vi "Compare.vi"() -> ()   [LabVIEW 2014]
doc: "Use this template to build a VI to use as a subVI."
uses:
  <vilib>/vision/NI_Vision_Development_Module.lvlib
panel:
  out "SrcA":T1(plugin-control)
  out "Dst":T1(plugin-control)
  # ":: MVi Framework V1.0 ::\nAuthor:Gaoke Yang\nEmail: gaoke.yang@yahoo.com\nWeb: www.mvicontrol.com\nCopyright (C) 2015, MVI Technologies All Rights Reserved"
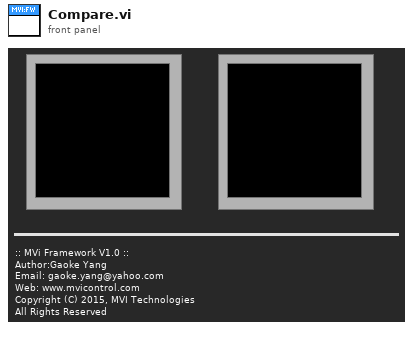
[diagram p1: front panel]
types:
  T1 = typedef "IMAQ Image.ctl" = refnum<image>
  T2 = typedef "Image Type" = u32
  T3 = enum32{"Average", "Min", "Max", "Clear  if < ", "Clear  if < or =", "Clear  if =", "Clear  if > or =", "Clear  if >"}
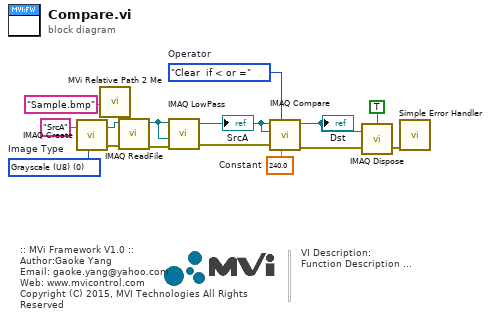
[diagram p0: block diagram]
diagram:
  w1 = T2 0 items=["Grayscale (U8)", "Grayscale (I16)", "Grayscale (SGL)", "Complex (CSG)", "RGB (U32)", "HSL (U32)", "RGB (U64)", "Grayscale (U16)"]  # Image Type
  w5 = sgl 240.0  # Constant
  w7 = T3."Clear  if < or ="  # Operator
  # "VI Description:\nFunction Description ..."
  # ":: MVi Framework V1.0 ::\nAuthor:Gaoke Yang\nEmail: gaoke.yang@yahoo.com\nWeb: www.mvicontrol.com\nCopyright (C) 2015, MVI Technologies All Rights Reserved"
  n1 = call "IMAQ Create"("Image Name"="SrcA" ("name or relative path"), "Image Type"=w1) -> ("New Image"=w10:T1, "error out"=w13:errorcluster)  [unwired: 2 in, 1 out]
  n2 = call "MVi Relative Path 2 Me.vi"("Relative Path"="Sample.bmp" ("name or relative path")) -> ("Appended Dir"=w11:path)  [unwired: 5 in, 1 out]
  n3 = call "IMAQ ReadFile"("File Path"=w11, "error in (no error)"=w13, "Image"=w10) -> ("error out"=w9:errorcluster, "Image Out"=w8:T1)  [unwired: 4 in, 3 out]
  n4 = call "IMAQ LowPass"("Image Src"=w8, "Image Dst"=w8, "error in (no error)"=w9) -> ("Image Dst Out"=w6:T1, "error out"=w2:errorcluster)  [unwired: 4 in]
  "SrcA" <- w6
  n5 = call "IMAQ Compare"("Constant"=w5, "Operator"=w7, "error in (no error)"=w2, "Image Dst"=w6, "Image Src A"=w6) -> ("error out"=w4:errorcluster, "Image Dst Out"=w3:T1)  [unwired: 5 in]
  "Dst" <- w3
  n6 = call "IMAQ Dispose"("All Images? (No)"=TRUE, "Image"=w3, "error in (no error)"=w4) -> ("error out"=w15:errorcluster)  [unwired: 3 out]
  n7 = call <vilib>:"Simple Error Handler.vi"("error in (no error)"=w15) -> ()  [unwired: 1 in, 8 out]
